vi "Read Table Infor.vi"(8 "error in (no error)":errorcluster, 11 "Abstruct Data Type in":refnum<class "Abstruct Data Type.lvclass">) -> (0 "error out":errorcluster, 2 "Table Infor":refnum<class "Data List.lvclass">[](array[class]), 3 "Abstruct Data Type out":refnum<class "Abstruct Data Type.lvclass">)   [LabVIEW 2020, in "Abstruct Data Type.lvclass"]
uses:
  Abstruct Data Type.lvclass
  Data List/Data List.lvclass
  Abstruct Data Type.lvclass/Abstruct Data Type.ctl
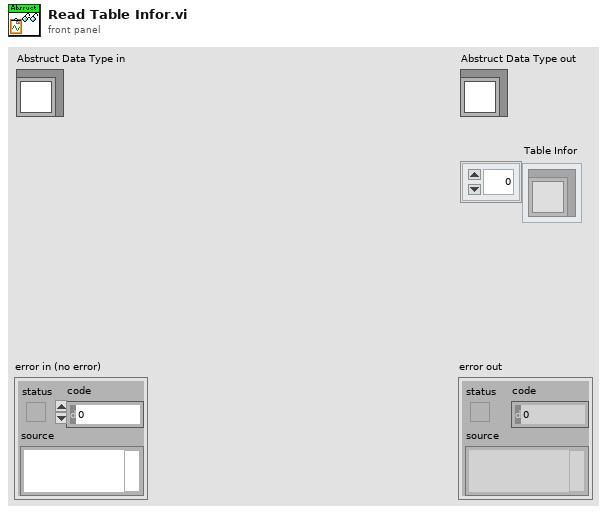
[diagram p1: front panel]
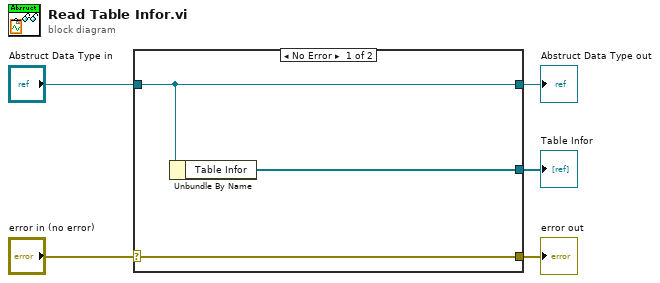
[diagram p0: block diagram]
diagram:
  n1 = case shown="No Error" "error in (no error)" {
    selector: "error in (no error)" -> [w8 w9]
    tunnel: [w8 w9] -> w4
    tunnel: [w7 w10] -> w2
    tunnel: "Abstruct Data Type in" -> [w7 w10]
    tunnel: [w6 _] -> w1
    frame No Error {
      n2 = Unbundle By Name(w7) -> ("Table Infor"=w6:refnum<class "Data List.lvclass">[])
    }
    frame Error {
    }
  }
  "error out" <- w4
  "Abstruct Data Type out" <- w2
  "Table Infor" <- w1
